vi "Example - Find Text.vi"() -> ()   [LabVIEW 2014]
doc: "This VI demonstrates how to call the Find Text VI."
panel:
  in  "String":string="The quick brown fox jumped over the lazy dog.  The quick brown fox jumped over the lazy dog.  The quick brown fox jumped over the lazy dog.  The quick brown fox jumped over the lazy dog.  The quick brown fox jumped over the lazy dog.  The quick brown fox jumped over the lazy dog.  The quick brown fox jumped over the lazy dog.  The quick brown fox jumped over the lazy dog.  The quick brown fox jumped over the lazy dog.  The quick brown fox jumped over the lazy dog.  The quick brown fox jumped over the lazy dog.  The quick brown fox jumped over the lazy dog.  The quick brown fox jumped over the lazy dog.  The quick brown fox jumped over the lazy dog.  The quick brown fox jumped over the lazy dog.  The quick brown fox jumped over the lazy dog.The quick brown fox jumped over the lazy dog.  The quick brown fox jumped over the lazy dog.  The quick brown fox jumped over the lazy dog.  The quick brown fox jumped over the lazy dog.  The quick brown fox jumped over the lazy dog.  The quick brown fox jumped over the lazy dog.  The quick brown fox jumped over the lazy dog.  The quick brown fox jumped over the lazy dog.The quick brown fox jumped over the lazy dog.  The quick brown fox jumped over the lazy dog.  The quick brown fox jumped over the lazy dog.  The quick brown fox jumped over the lazy dog.  The quick brown fox jumped over the lazy dog.  The quick brown fox jumped over the lazy dog.  The quick brown fox jumped over the lazy dog.  The quick brown fox jumped over the lazy dog.The quick brown fox jumped over the lazy dog.  The quick brown fox jumped over the lazy dog.  The quick brown fox jumped over the lazy dog.  The quick brown fox jumped over the lazy dog.  The quick brown fox jumped over the lazy dog.  The quick brown fox jumped over the lazy dog.  The quick brown fox jumped over the lazy dog.  The quick brown fox jumped over the lazy dog.The quick brown fox jumped over the lazy dog.  The quick brown fox jumped over the lazy dog.  The quick brown fox jumped over the lazy dog.  The quick brown fox jumped over the lazy dog.  The quick brown fox jumped over the lazy dog.  The quick brown fox jumped over the lazy dog.  The quick brown fox jumped over the lazy dog.  The quick brown fox jumped over the lazy dog.The quick brown fox jumped over the lazy dog.  The quick brown fox jumped over the lazy dog.  The quick brown fox jumped over the lazy dog.  The quick brown fox jumped over the lazy dog.  The quick brown fox jumped over the lazy dog.  The quick brown fox jumped over the lazy dog.  The quick brown fox jumped over the lazy dog.  The quick brown fox jumped over the lazy dog.The quick brown fox jumped over the lazy dog.  The quick brown fox jumped over the lazy dog.  The quick brown fox jumped over the lazy dog.  The quick brown fox jumped over the lazy dog.  The quick brown fox jumped over the lazy dog.  The quick brown fox jumped over the lazy dog.  The quick brown fox jumped over the lazy dog.  The quick brown fox jumped over the lazy dog.The quick brown fox jumped over the lazy dog.  The quick brown fox jumped over the lazy dog.  The quick brown fox jumped over the lazy dog.  The quick brown fox jumped over the lazy dog.  The quick brown fox jumped over the lazy dog.  The quick brown fox jumped over the lazy dog.  The quick brown fox jumped over the lazy dog.  The quick brown fox jumped over the lazy dog.The quick brown fox jumped over the lazy dog.  The quick brown fox jumped over the lazy dog.  The quick brown fox jumped over the lazy dog.  The quick brown fox jumped over the lazy dog.  The quick brown fox jumped over the lazy dog.  The quick brown fox jumped over the lazy dog.  The quick brown fox jumped over the lazy dog.  The quick brown fox jumped over the lazy dog.The quick brown fox jumped over the lazy dog.  The quick brown fox jumped over the lazy dog.  The quick brown fox jumped over the lazy dog.  The quick brown fox jumped over the lazy dog.  The quick brown fox jumped over the lazy dog.  The quick brown fox jumped over the lazy dog.  The quick brown fox jumped over the lazy dog.  The quick brown fox jumped over the lazy dog.The quick brown fox jumped over the lazy dog.  The quick brown fox jumped over the lazy dog.  The quick brown fox jumped over the lazy dog.  The quick brown fox jumped over the lazy dog.  The quick brown fox jumped over the lazy dog.  The quick brown fox jumped over the lazy dog.  The quick brown fox jumped over the lazy dog.  The quick brown fox jumped over the lazy dog.The quick brown fox jumped over the lazy dog.  The quick brown fox jumped over the lazy dog.  The quick brown fox jumped over the lazy dog.  The quick brown fox jumped over the lazy dog.  The quick brown fox jumped over the lazy dog.  The quick brown fox jumped over the lazy dog.  The quick brown fox jumped over the lazy dog.  The quick brown fox jumped over the lazy dog.The quick brown fox jumped over the lazy dog.  The quick brown fox jumped over the lazy dog.  The quick brown fox jumped over the lazy dog.  The quick brown fox jumped over the lazy dog.  The quick brown fox jumped over the lazy dog.  The quick brown fox jumped over the lazy dog.  The quick brown fox jumped over the lazy dog.  The quick brown fox jumped over the lazy dog.The quick brown fox jumped over the lazy dog.  The quick brown fox jumped over the lazy dog.  The quick brown fox jumped over the lazy dog.  The quick brown fox jumped over the lazy dog.  The quick brown fox jumped over the lazy dog.  The quick brown fox jumped over the lazy dog.  The quick brown fox jumped over the lazy dog.  The quick brown fox jumped over the lazy dog.The quick brown fox jumped over the lazy dog.  The quick brown fox jumped over the lazy dog.  The quick brown fox jumped over the lazy dog.  The quick brown fox jumped over the lazy dog.  The quick brown fox jumped over the lazy dog.  The quick brown fox jumped over the lazy dog.  The quick brown fox jumped over the lazy dog.  The quick brown fox jumped over the lazy dog.The quick brown fox jumped over the lazy dog.  The quick brown fox jumped over the lazy dog.  The quick brown fox jumped over the lazy dog.  The quick brown fox jumped over the lazy dog.  The quick brown fox jumped over the lazy dog.  The quick brown fox jumped over the lazy dog.  The quick brown fox jumped over the lazy dog.  The quick brown fox jumped over the lazy dog.The quick brown fox jumped over the lazy dog.  The quick brown fox jumped over the lazy dog.  The quick brown fox jumped over the lazy dog.  The quick brown fox jumped over the lazy dog.  The quick brown fox jumped over the lazy dog.  The quick brown fox jumped over the lazy dog.  The quick brown fox jumped over the lazy dog.  The quick brown fox jumped over the lazy dog.The quick brown fox jumped over the lazy dog.  The quick brown fox jumped over the lazy dog.  The quick brown fox jumped over the lazy dog.  The quick brown fox jumped over the lazy dog.  The quick brown fox jumped over the lazy dog.  The quick brown fox jumped over the lazy dog.  The quick brown fox jumped over the lazy dog.  The quick brown fox jumped over the lazy dog.The quick brown fox jumped over the lazy dog.  The quick brown fox jumped over the lazy dog.  The quick brown fox jumped over the lazy dog.  The quick brown fox jumped over the lazy dog.  The quick brown fox jumped over the lazy dog.  The quick brown fox jumped over the lazy dog.  The quick brown fox jumped over the lazy dog.  The quick brown fox jumped over the lazy dog."
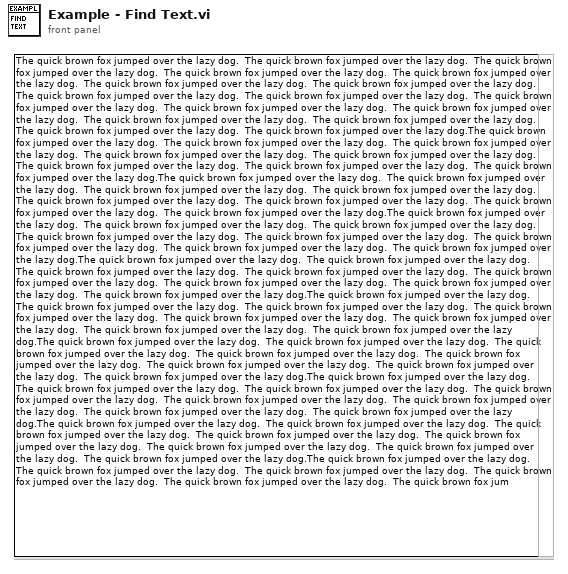
[diagram p1: front panel]
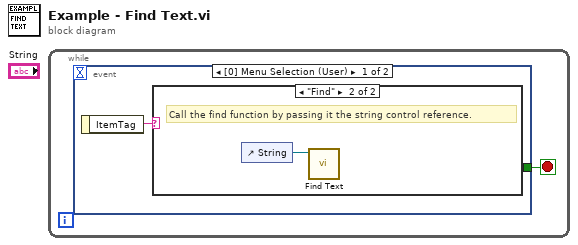
[diagram p0: block diagram]
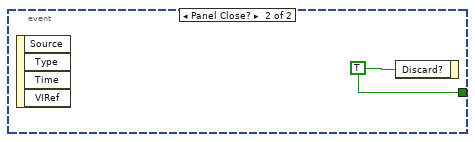
[diagram p3: hidden frame]
diagram:
  n1 = while {
    stop <- w1 stop-if-true
    n2 = event shown="[0] Menu Selection (User)" {
      selector: _ -> [_ _]
      dyn-events: _ -> [_ _]
      timeout: _ -> [_ _]
      tunnel: [_ w4] -> w1
      event Menu Selection (User) {
        n3 = event-data() -> ("ItemTag"=w2:string)  [unwired: 1 out]
        n4 = case shown="\"Find\"" w2 {
          frame Default {
          }
          frame "Find" {
            # "Call the find function by passing it the string control reference."
            n5 = control-ref of="String"() -> (w3:refnum<vi>)
            n6 = call "Find Text.vi"("String Reference"=w3) -> ()  [unwired: 1 in, 10 out]
          }
        }
      }
      event Panel Close? {
        w4 = TRUE ("Discard?")
        n7 = event-data() -> ()  [unwired: 5 out]
        n8 = event-data("Discard?"=w4) -> ()  [unwired: 1 in, 1 out]
      }
    }
  }
